vi "FVIR and LDO Modbus Checker.vi"() -> ()   [LabVIEW 2019]
uses:
  <vilib>/NI/Modbus Library/API/Wrapper/Create TCP Master.vi
  <vilib>/NI/Modbus Library/API/Master/Modbus Master.lvclass
  <vilib>/NI/Modbus Library/API/Wrapper/API Main.lvlib
panel:
  out "x-y 2":dbl
  out "x-y":dbl
  out "Outlet intellifaucet":u16
  out "Hot Water Inlet to Intellifaucet":u16
  out "Cold Water Inlet to Intellifaucet":u16
  out "Spare Thermocouple Input Type T":u16
  out "Ambient Air Temperature":u16
  out "Water Outlet - Temperature":u16
  out "Water Inlet - Temperature":u16
  in  "stop":bool
  out "Boolean array":bool[](array[boolean])
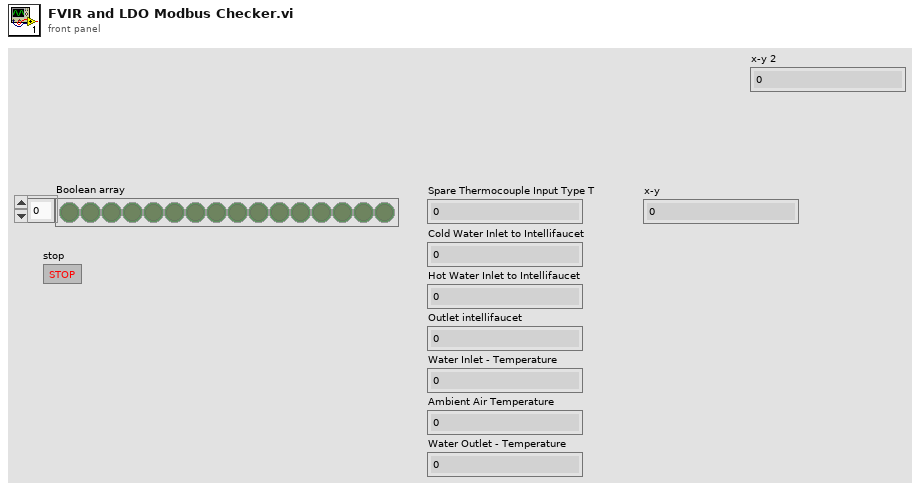
[diagram p1: front panel]
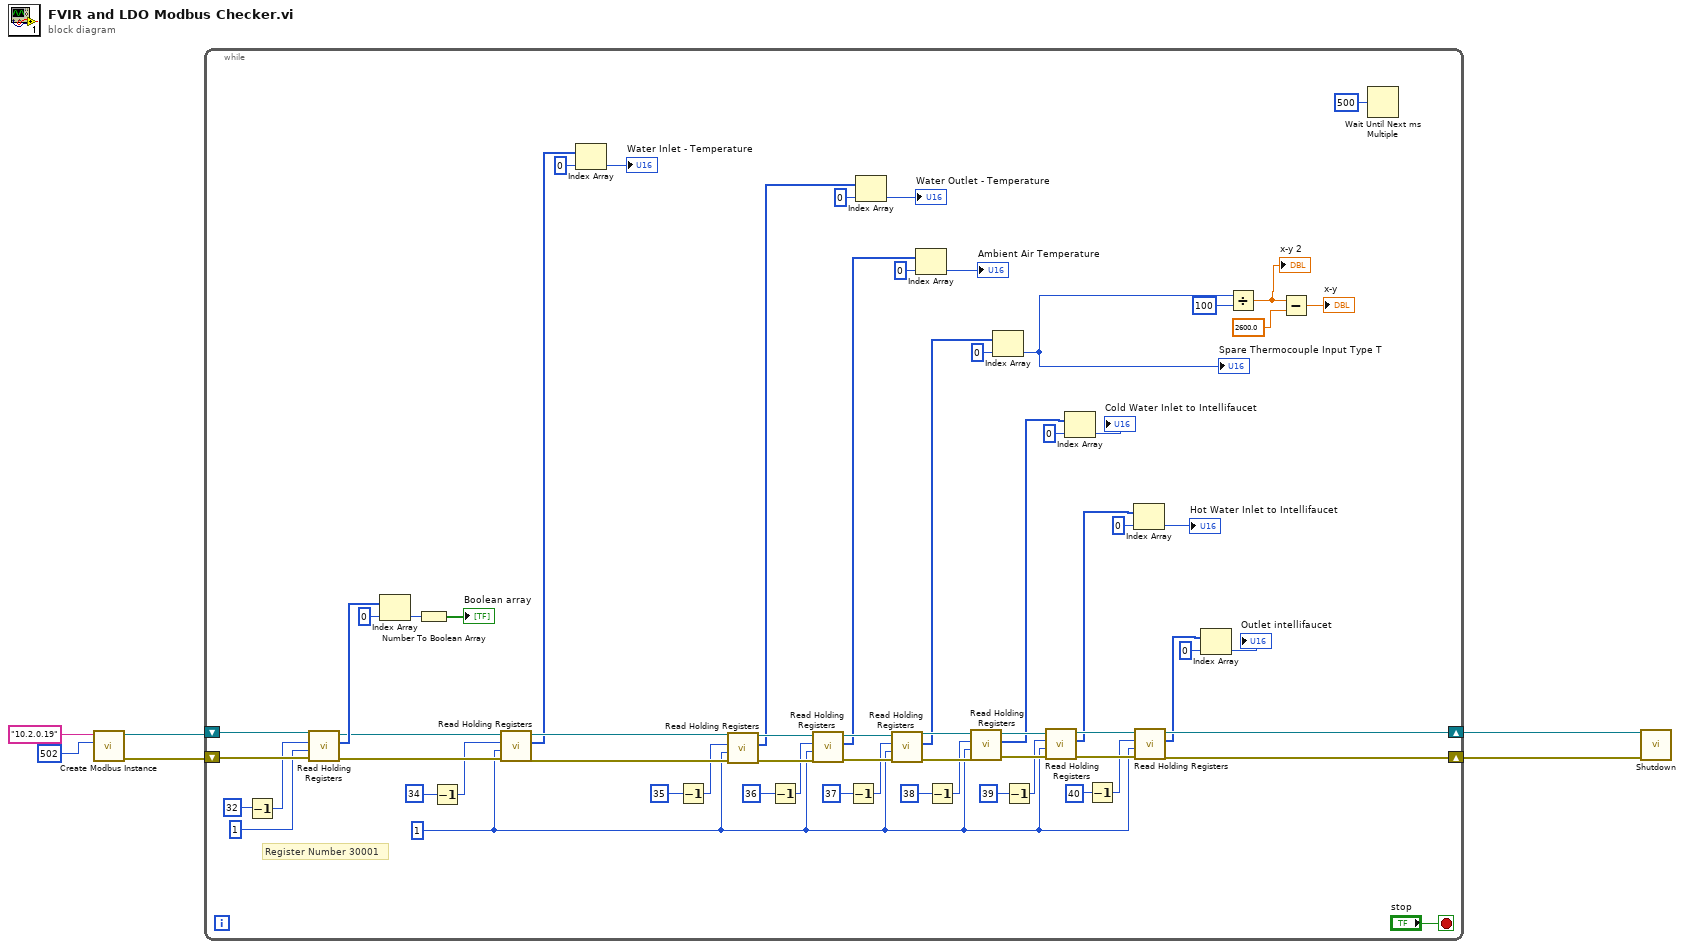
[diagram p0: block diagram]
diagram:
  n1 = call-poly <vilib>:"Create Modbus Instance.vi"("port (502)"=u16 502, "address"="10.2.0.19") -> ("error out"=w3:errorcluster, "TCP master instance"=w4:refnum<class "Modbus Master.lvclass">)  [unwired: 8 in]
  n2 = while {
    shift-right: [w50] -> w2
    shift-left: w4 -> [w73]
    shift-right: [w49] -> w1
    shift-left: w3 -> [w72]
    stop <- "stop" stop-if-true
    w21 = u16 1 ("number of inputs")
    # "Register Number 30001"
    n3 = Decrement(x=u16 32 ("starting address")) -> (x-1=w64:u16)
    n4 = call-dynamic "Read Holding Registers.vi"("error in"=w72, "number of inputs"=u16 1, "starting address"=w64, "Modbus master in"=w73) -> ("error out"=w63:errorcluster, "register values"=w70:u16[], "Modbus master out"=w66:refnum<class "Modbus Master.lvclass">)  [unwired: 5 in]
    n5 = Index Array(array=w70, index=0) -> (element=w68:u16)
    n6 = Number To Boolean Array(number=w68) -> (Boolean array=→"Boolean array":bool[])
    n7 = Decrement(x=u16 34 ("starting address")) -> (x-1=w19:u16)
    n8 = call-dynamic "Read Holding Registers.vi"("error in"=w63, "number of inputs"=w21, "starting address"=w19, "Modbus master in"=w66) -> ("error out"=w61:errorcluster, "register values"=w46:u16[], "Modbus master out"=w62:refnum<class "Modbus Master.lvclass">)  [unwired: 5 in]
    n9 = Index Array(array=w46, index=0) -> (element=→"Water Inlet - Temperature":u16)
    n10 = Decrement(x=u16 35 ("starting address")) -> (x-1=w17:u16)
    n11 = call-dynamic "Read Holding Registers.vi"("error in"=w61, "number of inputs"=w21, "starting address"=w17, "Modbus master in"=w62) -> ("error out"=w60:errorcluster, "register values"=w42:u16[], "Modbus master out"=w59:refnum<class "Modbus Master.lvclass">)  [unwired: 5 in]
    n12 = Decrement(x=u16 36 ("starting address")) -> (x-1=w15:u16)
    n13 = call-dynamic "Read Holding Registers.vi"("error in"=w60, "number of inputs"=w21, "starting address"=w15, "Modbus master in"=w59) -> ("error out"=w57:errorcluster, "register values"=w39:u16[], "Modbus master out"=w58:refnum<class "Modbus Master.lvclass">)  [unwired: 5 in]
    n14 = Decrement(x=u16 37 ("starting address")) -> (x-1=w13:u16)
    n15 = Index Array(array=w42, index=0) -> (element=→"Water Outlet - Temperature":u16)
    n16 = call-dynamic "Read Holding Registers.vi"("error in"=w57, "number of inputs"=w21, "starting address"=w13, "Modbus master in"=w58) -> ("error out"=w56:errorcluster, "register values"=w36:u16[], "Modbus master out"=w55:refnum<class "Modbus Master.lvclass">)  [unwired: 5 in]
    n17 = Index Array(array=w39, index=0) -> (element=→"Ambient Air Temperature":u16)
    n18 = Decrement(x=u16 38 ("starting address")) -> (x-1=w11:u16)
    n19 = call-dynamic "Read Holding Registers.vi"("error in"=w56, "number of inputs"=w21, "starting address"=w11, "Modbus master in"=w55) -> ("error out"=w53:errorcluster, "register values"=w34:u16[], "Modbus master out"=w54:refnum<class "Modbus Master.lvclass">)  [unwired: 5 in]
    n20 = Index Array(array=w36, index=0) -> (element=w26:u16)
    "Spare Thermocouple Input Type T" <- w26
    n21 = Decrement(x=u16 39 ("starting address")) -> (x-1=w9:u16)
    n22 = call-dynamic "Read Holding Registers.vi"("error in"=w53, "number of inputs"=w21, "starting address"=w9, "Modbus master in"=w54) -> ("error out"=w52:errorcluster, "register values"=w31:u16[], "Modbus master out"=w51:refnum<class "Modbus Master.lvclass">)  [unwired: 5 in]
    n23 = Index Array(array=w34, index=0) -> (element=→"Cold Water Inlet to Intellifaucet":u16)
    n24 = Decrement(x=u16 40 ("starting address")) -> (x-1=w8:u16)
    n25 = Index Array(array=w31, index=0) -> (element=→"Hot Water Inlet to Intellifaucet":u16)
    n26 = call-dynamic "Read Holding Registers.vi"("error in"=w52, "number of inputs"=w21, "starting address"=w8, "Modbus master in"=w51) -> ("error out"=w49:errorcluster, "register values"=w28:u16[], "Modbus master out"=w50:refnum<class "Modbus Master.lvclass">)  [unwired: 5 in]
    n27 = Index Array(array=w28, index=0) -> (element=→"Outlet intellifaucet":u16)
    n28 = Divide(x=w26, y=u16 100) -> (x/y=w22:dbl)
    "x-y 2" <- w22
    n29 = Subtract(x=w22, y=2600.0) -> (x-y=→"x-y":dbl)
    n30 = Wait Until Next ms Multiple(millisecond multiple=u32 500) -> ()  [unwired: 1 out]
  }
  n31 = call-dynamic "Shutdown.vi"("error in"=w1, "Modbus master in"=w2) -> ()  [unwired: 9 in, 1 out]
